vi "TEST.vi"() -> ()   [LabVIEW 2017]
uses:
  <vilib>/Platform/TimedLoop/XDataNode/wakeup.ctl
  <vilib>/Platform/TimedLoop/XDataNode/XDNodeRunTimeDep.lvlib
  <vilib>/Platform/TimedLoop/XDataNode/nitl_modes.ctl
  <vilib>/Platform/TimedLoop/XDataNode/timing_clust.ctl
  <vilib>/Platform/TimedLoop/XDataNode/XDataNode.xnode
  <vilib>/eio/EIONode/EIONode.xnode
  <vilib>/rvi/eio/common/nirviEmuTemplateMethod_errors.vi
panel:
  in  "Filter On":bool=TRUE
  in  "stop":bool
  in  "Numeric":i16
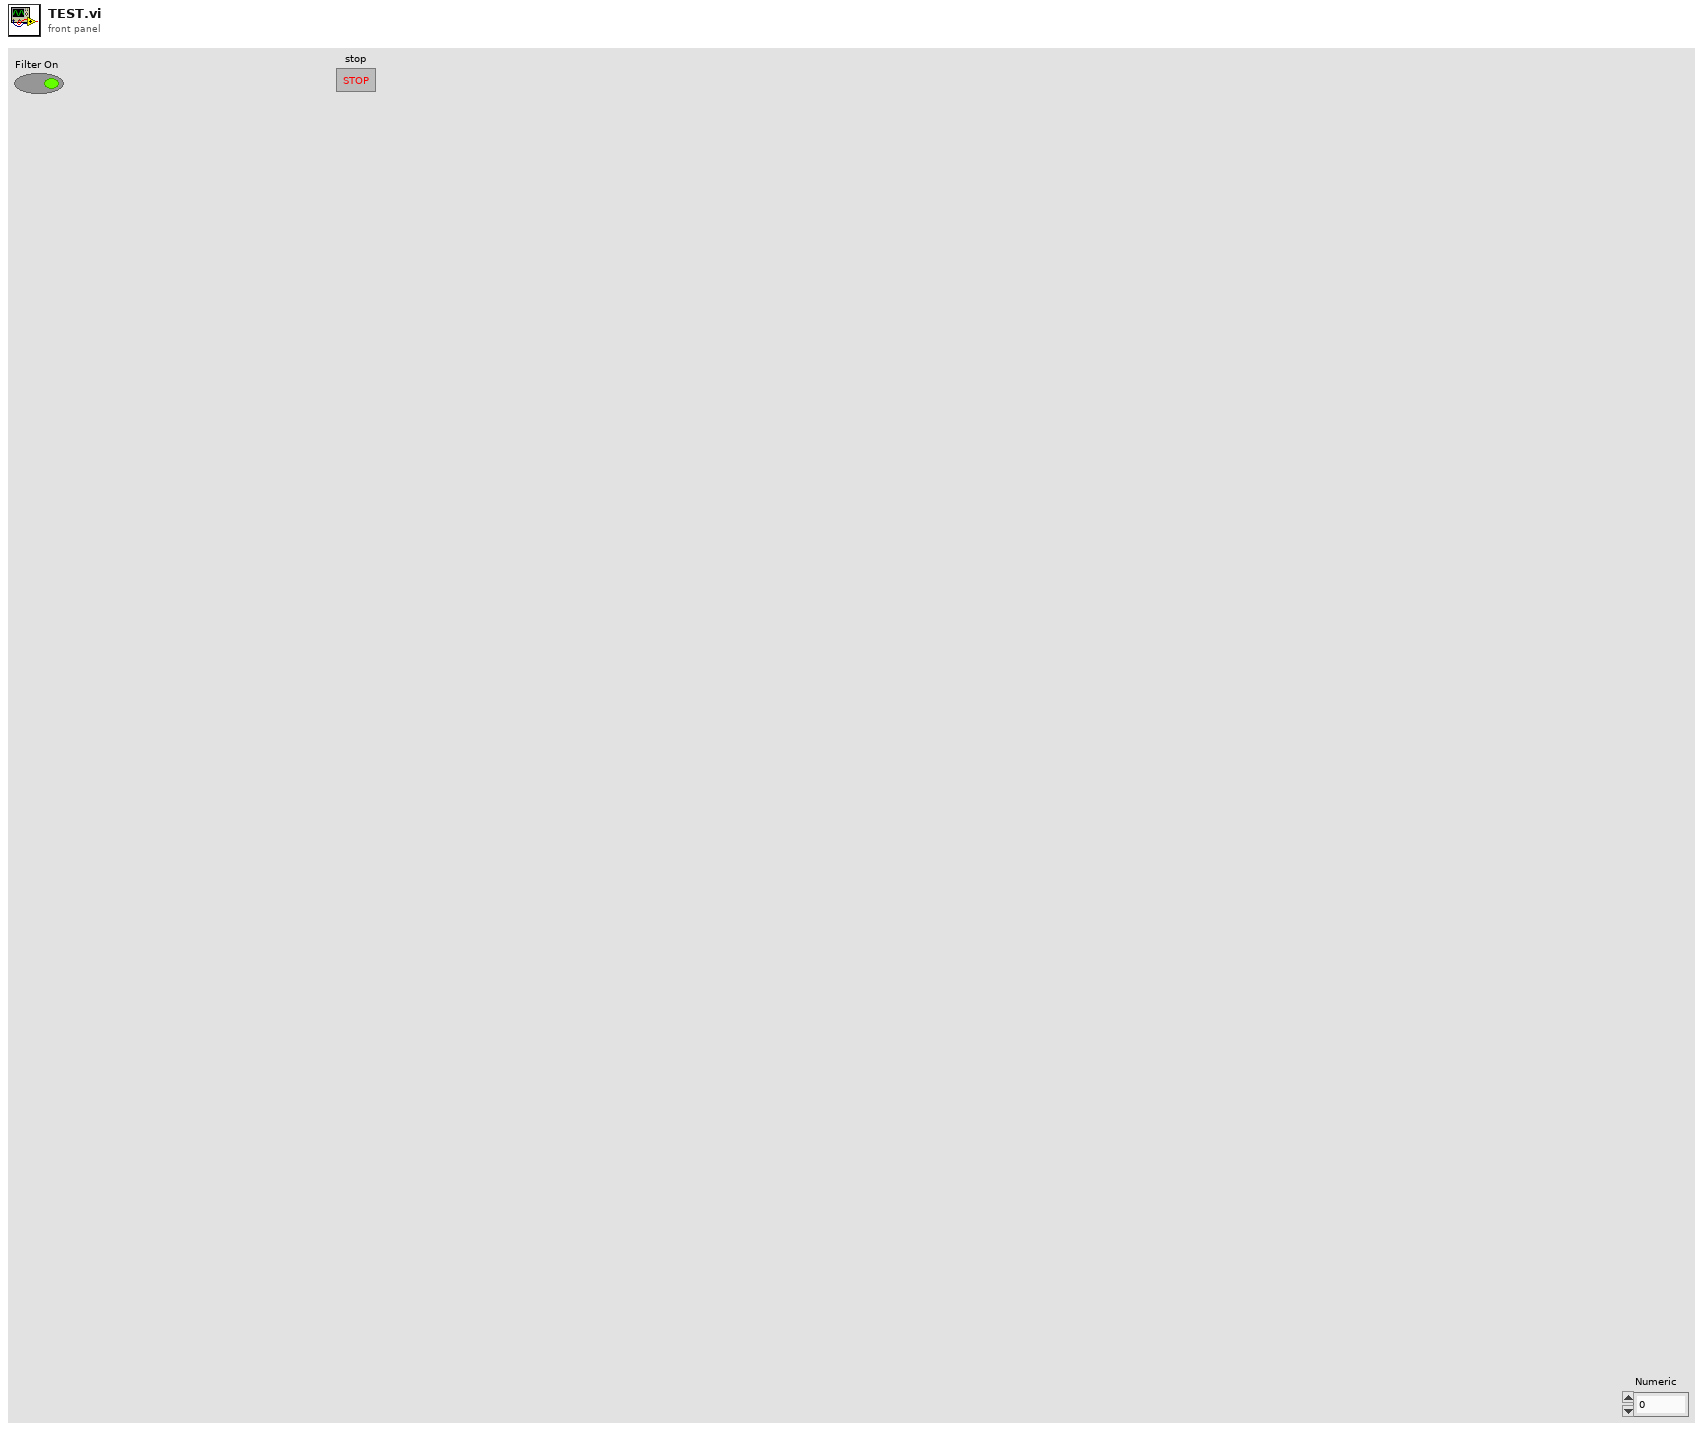
[diagram p1: front panel]
types:
  T1 = typedef "XDNodeRunTimeDep.lvlib/timing_clust.ctl" = cluster{"Expected End [f-1]":u64, "Actual End [f-1]":u64, "Finished Late? [f-1]":bool, "Expected End [i-1]":u64, "Actual End [i-1]":u64, "Finished Late? [i-1]":bool, "Expected Start [i]":u64, "Actual Start [i]":u64, "Expected Start [f]":u64, "Actual Start [f]":u64, "Source Name":string, "Structure Name":string, "Period":i64, "Deadline":i64, "Offset":i64, "Start":i64, "Priority":i32, "Timeout":i32, "Mode":T2, "Wakeup Reason":T3, "Error":errorcluster, "Source Type":string, "Secondary Source Type":string, "Global End Time":u64, "Global Start Time":u64, "Frame Duration":u64, "Iteration Duration":u64, "Assigned CPU":i32, "I/O Scan Engine Mode":u32}
  T2 = typedef "XDNodeRunTimeDep.lvlib/nitl_modes.ctl" = enum32{"No Change", "Process missed periods, maintain original phase", "Discard missed periods, maintain original phase", "Process missed periods, ignore original phase", "Discard missed periods, ignore original phase"}
  T3 = typedef "XDNodeRunTimeDep.lvlib/wakeup.ctl" = enum32{"Normal", "Aborted", "Asynchronous wakeup", "Timing source error", "Timed loop error", "Timeout"}
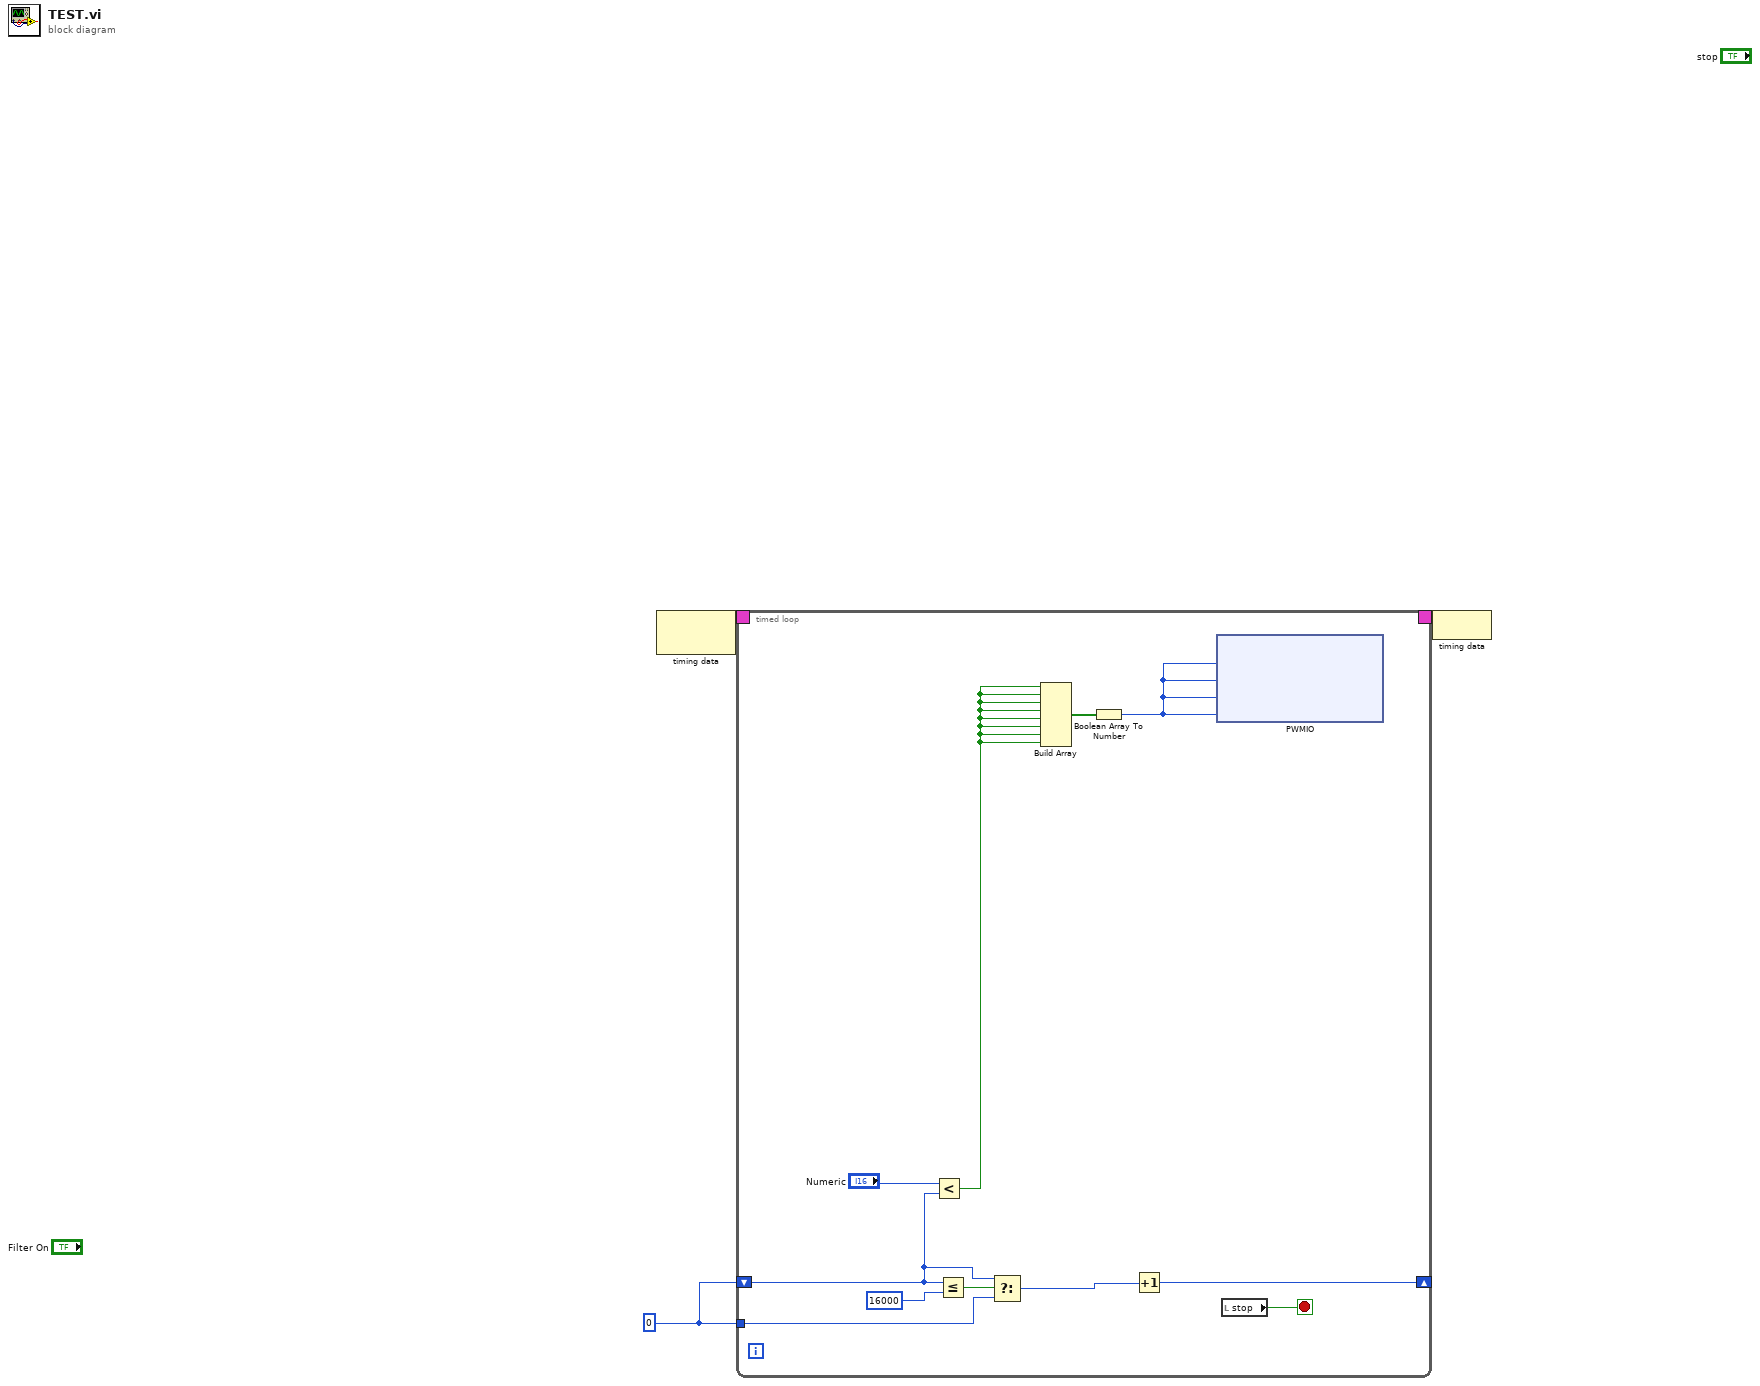
[diagram p0: block diagram]
diagram:
  w1 = i16 0 ("Numeric")
  n1 = node-c288() -> (w3:T1)  [unwired: 1 in]
  n2 = timed-loop {
    timing: w3 -> [_]
    timing-out: [_] -> w2
    shift-right: [w11] -> _
    shift-left: w1 -> [w6]
    tunnel: w1 -> [w10]
    stop <- w13 stop-if-true
    n3 = Less?(x="Numeric", y=w6) -> (x < y?=w5:bool)
    n4 = Less Or Equal?(x=w6, y=i16 16000 ("Period")) -> (x <= y?=w4:bool)
    n5 = Select(t=w6, s=w4, f=w10) -> (s? t:f=w12:i16)
    n6 = Build Array(w5, w5, w5, w5, w5, w5, w5, w5) -> (w9:bool[])
    n7 = Boolean Array To Number(Boolean array=w9) -> (number=w8:u8)
    n8 = Increment(x=w12) -> (x+1=w11:i16)
    n9 = xnode ("PWMIO")("Connector0/DIOPORT0"=w8, "Connector0/DIOPORT1"=w8, "Connector0/DIOPORT2"=w8, "Connector0/DIOPORT3"=w8) -> ()  [unwired: 4 in, 4 out]
    n10 = local read "stop"() -> (w13:bool)
  }
  n11 = node-c288(w2) -> ()
